vi "linear interpolation iiii- complex.vi"(0 "Array":cdb[](array[numeric]), 11 "center":i32=-1) -> (2 "sigma":dbl, 3 "directed sigma":dbl, 4 "left":cdb, 6 "center":cdb, 8 "right":cdb, 10 "mean":cdb, 12 "intercept":cdb, 14 "slope":cdb, 15 "interpolated average":cdb)   [LabVIEW 2018]
panel:
  out "sum z_n":cdb
  out "sum n z_n":cdb
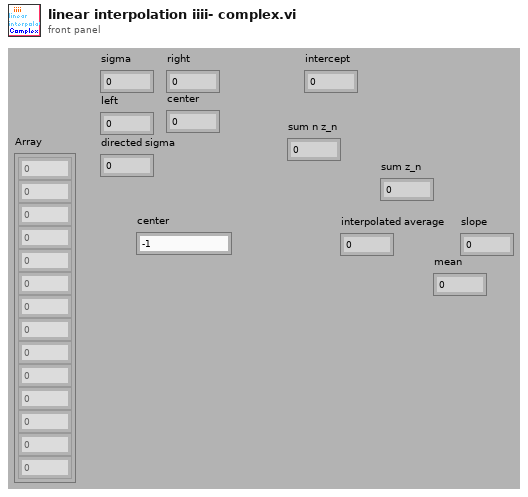
[diagram p1: front panel]
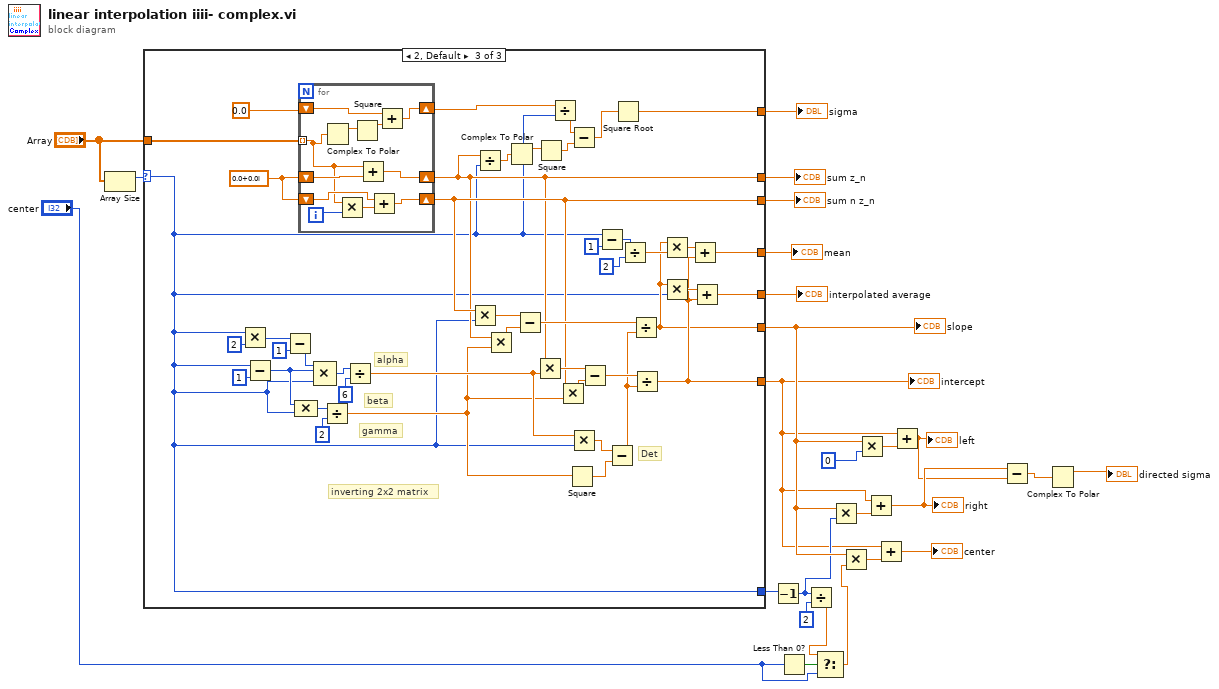
[diagram p0: block diagram]
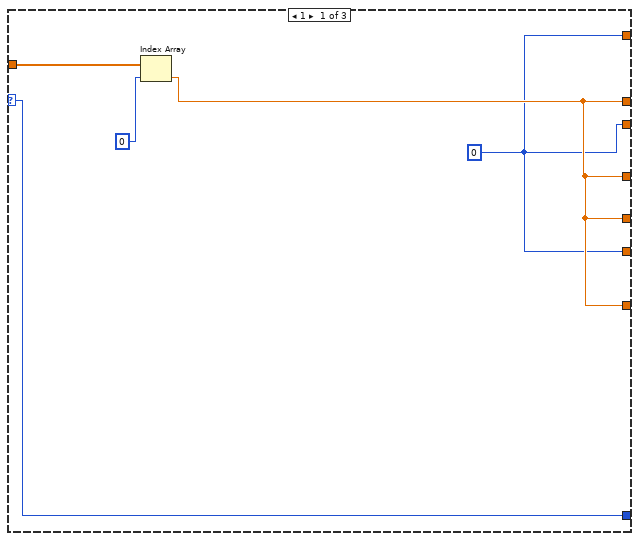
[diagram p2: hidden frame]
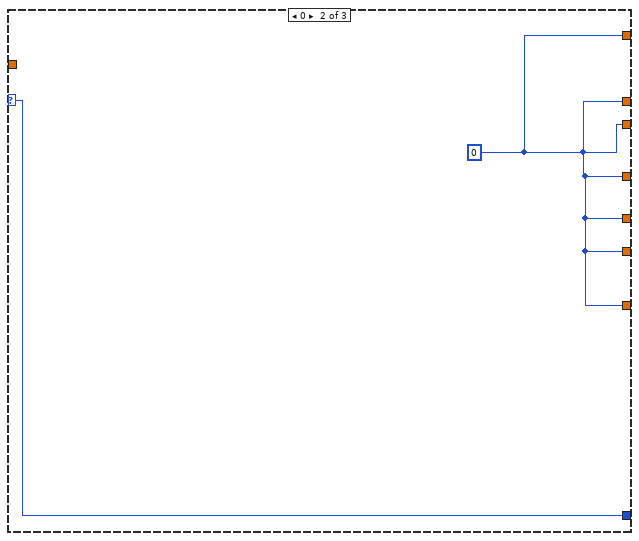
[diagram p3: hidden frame]
diagram:
  n1 = Array Size(array="Array") -> (size(s)=w20:i32)
  n2 = case shown="2, Default" w20 {
    selector: w20 -> [w26 w31 w38]
    tunnel: [w28 w32 w49] -> w9
    tunnel: [w27 w32 w48] -> w12
    tunnel: [w28 w32 w47] -> w25
    tunnel: [w28 w32 w46] -> w24
    tunnel: [w28 w32 w39] -> w23
    tunnel: [w27 w32 w45] -> w22
    tunnel: "Array" -> [w30 _ w44]
    tunnel: [w27 w32 w42] -> w19
    tunnel: [w26 w31 w38] -> w13
    frame 1 {
      w27 = 0 ("index")
      n3 = Index Array(array=w30, index=0) -> (element=w28:cdb)
    }
    frame 0 {
      w32 = 0 ("index")
    }
    frame 2, Default {
      w43 = cdb 0.0+0.0i
      # "inverting 2x2 matrix"
      # "Det"
      # "beta"
      # "gamma"
      # "alpha"
      n4 = Multiply(x=w38, y=2 ("n")) -> (x*y=w73:i32)
      n5 = Subtract(x=w38, y=1 ("n")) -> (x-y=w69:i32)
      n6 = Subtract(x=w73, y=1 ("n")) -> (x-y=w72:i32)
      n7 = Compound Arithmetic op=MULTIPLY(w69, w38) -> (w67:i32)
      n8 = for {
        tunnel: w44 -> [w79] mode=indexing
        shift-right: [w87] -> w39
        shift-left: w43 -> [w86]
        shift-right: [w84] -> w45
        shift-left: w43 -> [w82]
        shift-right: [w81] -> w41
        shift-left: 0.0 -> [w80]
        i -> [w83]
        n9 = Complex To Polar(r * e^(i*theta)=w79) -> (r=w78:dbl)  [unwired: 1 out]
        n10 = Multiply(x=w79, y=w83) -> (x*y=w85:cdb)
        n11 = Square(x=w78) -> (x^2=w77:dbl)
        n12 = Add(x=w79, y=w86) -> (x+y=w87:cdb)
        n13 = Add(x=w82, y=w85) -> (x+y=w84:cdb)
        n14 = Add(x=w80, y=w77) -> (x+y=w81:dbl)
      }
      n15 = Compound Arithmetic op=MULTIPLY(w72, w69, w38) -> (w71:i32)
      n16 = Divide(x=w67, y=2 ("n")) -> (x/y=w58:dbl)
      n17 = Divide(x=w71, y=6 ("n")) -> (x/y=w59:dbl)
      n18 = Multiply(x=w45, y=w38) -> (x*y=w63:cdb)
      n19 = Divide(x=w39, y=w38) -> (x/y=w36:cdb)
      n20 = Multiply(x=w39, y=w58) -> (x*y=w64:cdb)
      n21 = Complex To Polar(r * e^(i*theta)=w36) -> (r=w37:dbl)  [unwired: 1 out]
      n22 = Subtract(x=w63, y=w64) -> (x-y=w62:cdb)
      n23 = Multiply(x=w39, y=w59) -> (x*y=w60:cdb)
      n24 = Square(x=w37) -> (x^2=w34:dbl)
      n25 = Divide(x=w41, y=w38) -> (x/y=w35:dbl)
      n26 = Multiply(x=w45, y=w58) -> (x*y=w61:cdb)
      n27 = Square(x=w58) -> (x^2=w65:dbl)
      n28 = Subtract(x=w35, y=w34) -> (x-y=w33:dbl)
      n29 = Multiply(x=w59, y=w38) -> (x*y=w66:dbl)
      n30 = Subtract(x=w60, y=w61) -> (x-y=w57:cdb)
      n31 = Subtract(x=w38, y=1 ("n")) -> (x-y=w54:i32)
      n32 = Subtract(x=w66, y=w65) -> (x-y=w56:dbl)
      n33 = Square Root(x=w33) -> (sqrt(x)=w42:dbl)
      n34 = Divide(x=w54, y=2 ("n")) -> (x/y=w52:dbl)
      n35 = Divide(x=w62, y=w56) -> (x/y=w48:cdb)
      n36 = Divide(x=w57, y=w56) -> (x/y=w49:cdb)
      n37 = Multiply(x=w48, y=w52) -> (x*y=w51:cdb)
      n38 = Multiply(x=w48, y=w38) -> (x*y=w50:cdb)
      n39 = Add(x=w51, y=w49) -> (x+y=w46:cdb)
      n40 = Add(x=w50, y=w49) -> (x+y=w47:cdb)
    }
  }
  "interpolated average" <- w25
  "slope" <- w12
  "mean" <- w24
  "intercept" <- w9
  "sum n z_n" <- w22
  "sum z_n" <- w23
  "sigma" <- w19
  n41 = Decrement(x=w13) -> (x-1=w11:i32)
  n42 = Less Than 0?(x="center") -> (x < 0?=w8:bool)
  n43 = Divide(x=w11, y=2 ("n")) -> (x/y=w7:dbl)
  n44 = Select(t=w7, s=w8, f="center") -> (s? t:f=w5:dbl)
  n45 = Multiply(x=w12, y=w11) -> (x*y=w16:cdb)
  n46 = Multiply(x=w12, y=w5) -> (x*y=w15:cdb)
  n47 = Multiply(x=w12, y=0 ("n")) -> (x*y=w17:cdb)
  n48 = Add(x=w9, y=w16) -> (x+y=w4:cdb)
  "right" <- w4
  n49 = Add(x=w9, y=w15) -> (x+y=→"center":cdb)
  n50 = Add(x=w9, y=w17) -> (x+y=w3:cdb)
  "left" <- w3
  n51 = Subtract(x=w4, y=w3) -> (x-y=w2:cdb)
  n52 = Complex To Polar(r * e^(i*theta)=w2) -> (r=→"directed sigma":dbl)  [unwired: 1 out]
